vi "FestoCPX.Station.Prod.TakeAB.vi"(7 "SuckerID":i32, 8 "error in":errorcluster) -> (0 "error out":errorcluster, 1 "Slot":cluster{"A":bool, "B":bool}, 2 "Error reason B":T2, 3 "Error reason A":T2, 4 "Prod Present":T1)   [LabVIEW 2016]
uses:
  Sequence/Sequence.Test.BreakReason.ctl
  FestoCPX.Station.ProdPresent.ctl
  Station/Station.ValvePosition.ctl
  Station/Station.ProductSlot.ctl
  FestoCPX.Station.ProdArmPosition.ctl
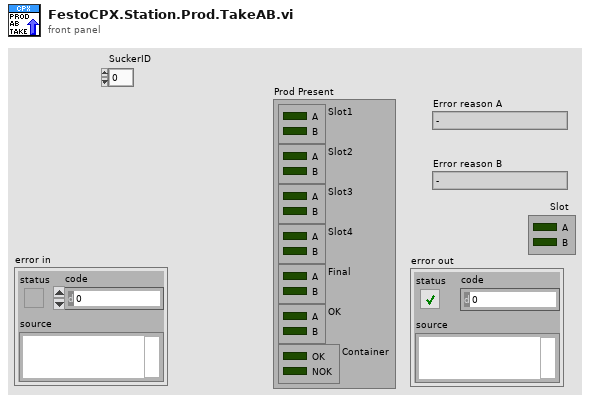
[diagram p1: front panel]
types:
  T1 = typedef "FestoCPX.Station.ProdPresent.ctl" = cluster{"Slot1":cluster{"A":bool, "B":bool}, "Slot2":cluster{"A":bool, "B":bool}, "Slot3":cluster{"A":bool, "B":bool}, "Slot4":cluster{"A":bool, "B":bool}, "Final":cluster{"A":bool, "B":bool}, "OK":cluster{"A":bool, "B":bool}, "Container":cluster{"OK":bool, "NOK":bool}}
  T2 = typedef "Sequence.Test.BreakReason.ctl" = enum16{"-", "NOK container", "OK container", "Rev empty", "Rev missing", "Rev wrong", "Fork missing", "Fork wrong", "NOK limit", "Unload failure", "Single slot", "Part done", "Err: Prod move work", "Err: Prod move home", "Err: Prod lift work", "Err: Prod lift home", "Err: Prod Arm Work", "Err: Prod Arm NOK", "Err: Prod Arm OK", "Err: Prod NOK suck", "Err: Prod NOK drop", "Err: Prod OK missing", "Err: Prod OK suck", "Err: Prod OK drop"}
  T3 = typedef "Station.ProductSlot.ctl" = enum8{"A", "B"}
  T4 = typedef "Station.ValvePosition.ctl" = enum16{"Home", "Work"}
  T5 = typedef "FestoCPX.Station.ProdArmPosition.ctl" = enum16{"Work", "OK", "NOK"}
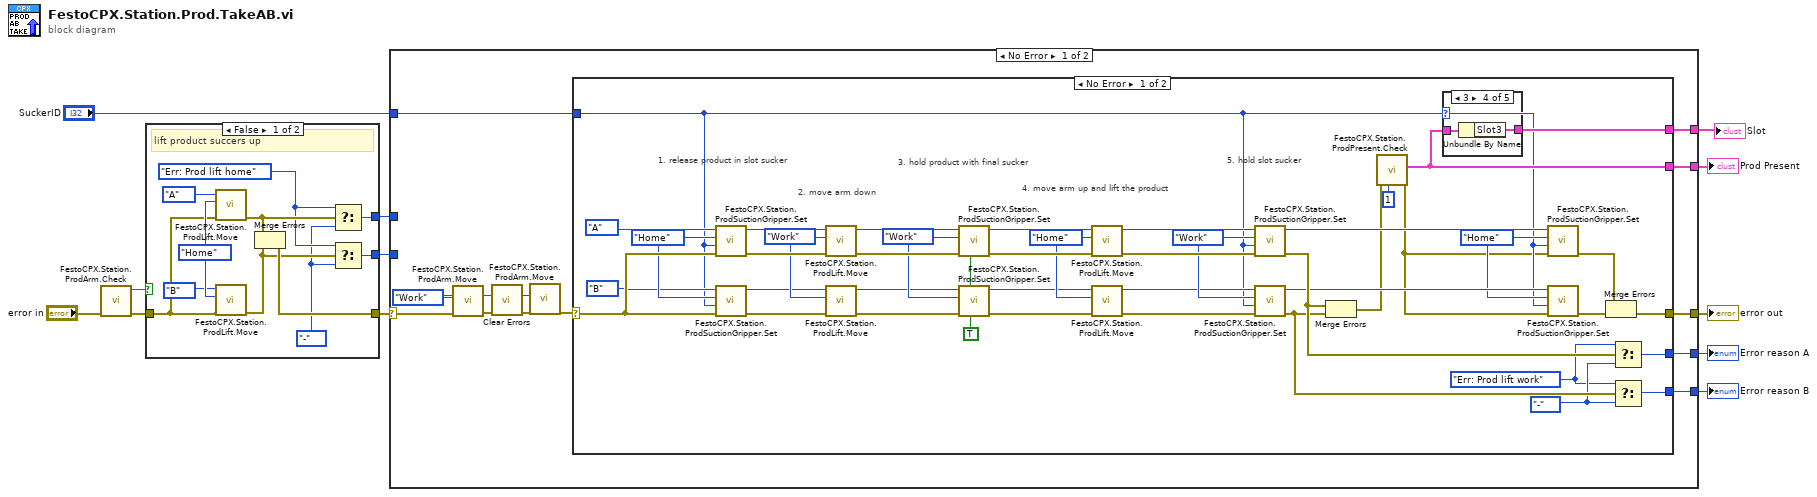
[diagram p0: block diagram]
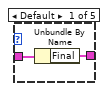
[diagram p2: hidden frame]
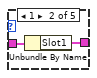
[diagram p3: hidden frame]
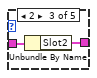
[diagram p4: hidden frame]
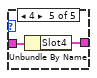
[diagram p5: hidden frame]
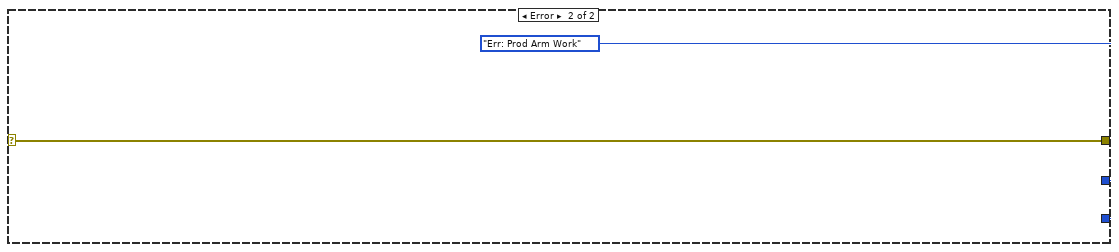
[diagram p6: hidden frame]
diagram:
  n1 = call "FestoCPX.Station.ProdArm.Check.vi"("error in"="error in") -> ("error out"=w12:errorcluster, "Work"=w11:bool)  [unwired: 6 in, 3 out]
  n2 = case shown="False" w11 {
    tunnel: w12 -> [w20 w24]
    tunnel: [w19 w24] -> w6
    tunnel: [w14 _] -> w10
    tunnel: [w13 _] -> w9
    frame False {
      w15 = Sequence.Test.BreakReason."-" ("Pause status")
      w16 = Sequence.Test.BreakReason."Err: Prod lift home" ("Pause status")
      w22 = Station.ValvePosition."Home" ("Position")
      # "lift product succers up"
      n3 = call "FestoCPX.Station.ProdLift.Move.vi"("error in"=w20, "Position"=w22, "Slot"=Station.ProductSlot."A") -> ("error out"=w18:errorcluster)  [unwired: 8 in]
      n4 = call "FestoCPX.Station.ProdLift.Move.vi"("error in"=w20, "Position"=w22, "Slot"=Station.ProductSlot."B") -> ("error out"=w17:errorcluster)  [unwired: 8 in]
      n5 = Merge Errors(w18, w17) -> (w19:errorcluster)
      n6 = Select(t=w16, s=w18, f=w15) -> (s? t:f=w14:T2)
      n7 = Select(t=w16, s=w17, f=w15) -> (s? t:f=w13:T2)
    }
    frame True {
      # "Arm already in work position"
    }
  }
  n8 = case shown="No Error" w6 {
    selector: w6 -> [w34 w81]
    tunnel: w10 -> [_ w83]
    tunnel: w9 -> [_ w82]
    tunnel: [w35 w83] -> w8
    tunnel: [w33 w82] -> w5
    tunnel: [w32 w81] -> w4
    tunnel: "SuckerID" -> [w31 _]
    tunnel: [w30 _] -> w2
    tunnel: [w29 _] -> w1
    frame No Error {
      w25 = FestoCPX.Station.ProdArmPosition."Work" ("Product Status")
      n9 = call "FestoCPX.Station.ProdArm.Move.vi"("error in"=w34, "Product Status"=w25) -> ("error out"=w28:errorcluster)  [unwired: 9 in]
      n10 = call <vilib>:"Clear Errors.vi"("error in (no error)"=w28) -> ("error out"=w27:errorcluster)  [unwired: 5 in, 1 out]
      n11 = call "FestoCPX.Station.ProdArm.Move.vi"("error in"=w27, "Product Status"=w25) -> ("error out"=w26:errorcluster)  [unwired: 9 in]
      n12 = case shown="No Error" w26 {
        selector: w26 -> [w62 w80]
        tunnel: [w51 w79] -> w35
        tunnel: [w52 w79] -> w33
        tunnel: [w40 w80] -> w32
        tunnel: w31 -> [w38 _]
        tunnel: [w48 _] -> w30
        tunnel: [w45 _] -> w29
        frame No Error {
          w39 = Station.ValvePosition."Home" ("Position")
          w46 = Sequence.Test.BreakReason."Err: Prod lift work" ("Pause status")
          w47 = Sequence.Test.BreakReason."-" ("Pause status")
          w54 = Station.ValvePosition."Work" ("Position")
          w57 = TRUE ("wait for product (F)")
          w59 = Station.ValvePosition."Work" ("Position")
          w61 = Station.ValvePosition."Home" ("Position")
          w58 = Station.ValvePosition."Home" ("Position")
          w60 = Station.ValvePosition."Work" ("Position")
          w43 = Station.ProductSlot."B" ("Slot")
          w44 = Station.ProductSlot."A" ("Slot")
          # "5. hold slot sucker"
          # "2. move arm down"
          # "4. move arm up and lift the product"
          # "3. hold product with final sucker"
          # "1. release product in slot sucker"
          n13 = call "FestoCPX.Station.ProdSuctionGripper.Set.vi"("error in"=w62, "Sucker (0: Final)"=w38, "Position"=w61, "Slot"=w44) -> ("error out"=w66:errorcluster)  [unwired: 6 in, 1 out]
          n14 = call "FestoCPX.Station.ProdSuctionGripper.Set.vi"("error in"=w62, "Sucker (0: Final)"=w38, "Position"=w61, "Slot"=w43) -> ("error out"=w65:errorcluster)  [unwired: 6 in, 1 out]
          n15 = call "FestoCPX.Station.ProdLift.Move.vi"("error in"=w66, "Position"=w60, "Slot"=w44) -> ("error out"=w67:errorcluster)  [unwired: 8 in]
          n16 = call "FestoCPX.Station.ProdLift.Move.vi"("error in"=w65, "Position"=w60, "Slot"=w43) -> ("error out"=w64:errorcluster)  [unwired: 8 in]
          n17 = call "FestoCPX.Station.ProdSuctionGripper.Set.vi"("wait for product (F)"=w57, "error in"=w67, "Position"=w59, "Slot"=w44) -> ("error out"=w68:errorcluster)  [unwired: 6 in, 1 out]
          n18 = call "FestoCPX.Station.ProdSuctionGripper.Set.vi"("wait for product (F)"=w57, "error in"=w64, "Position"=w59, "Slot"=w43) -> ("error out"=w63:errorcluster)  [unwired: 6 in, 1 out]
          n19 = call "FestoCPX.Station.ProdLift.Move.vi"("error in"=w68, "Position"=w58, "Slot"=w44) -> ("error out"=w56:errorcluster)  [unwired: 8 in]
          n20 = call "FestoCPX.Station.ProdLift.Move.vi"("error in"=w63, "Position"=w58, "Slot"=w43) -> ("error out"=w55:errorcluster)  [unwired: 8 in]
          n21 = call "FestoCPX.Station.ProdSuctionGripper.Set.vi"("error in"=w56, "Sucker (0: Final)"=w38, "Position"=w54, "Slot"=w44) -> ("error out"=w50:errorcluster)  [unwired: 6 in, 1 out]
          n22 = call "FestoCPX.Station.ProdSuctionGripper.Set.vi"("error in"=w55, "Sucker (0: Final)"=w38, "Position"=w54, "Slot"=w43) -> ("error out"=w49:errorcluster)  [unwired: 6 in, 1 out]
          n23 = Merge Errors(w50, w49) -> (w36:errorcluster)
          n24 = call "FestoCPX.Station.ProdPresent.Check.vi"("Stab Counter (0)"=1 ("Max Stab time [ms] (0)"), "error in"=w36) -> ("error out"=w37:errorcluster, "Prod Present"=w48:T1)  [unwired: 4 in, 4 out]
          n25 = case shown="3" w38 {
            tunnel: w48 -> [w70 w72 w74 w76 w78]
            tunnel: [w69 w71 w73 w75 w77] -> w45
            frame Default {
              n26 = Unbundle By Name(w70) -> ("Final"=w69:cluster{"A":bool, "B":bool})
            }
            frame 1 {
              n27 = Unbundle By Name(w72) -> ("Slot1"=w71:cluster{"A":bool, "B":bool})
            }
            frame 2 {
              n28 = Unbundle By Name(w74) -> ("Slot2"=w73:cluster{"A":bool, "B":bool})
            }
            frame 3 {
              n29 = Unbundle By Name(w76) -> ("Slot3"=w75:cluster{"A":bool, "B":bool})
            }
            frame 4 {
              n30 = Unbundle By Name(w78) -> ("Slot4"=w77:cluster{"A":bool, "B":bool})
            }
          }
          n31 = call "FestoCPX.Station.ProdSuctionGripper.Set.vi"("error in"=w37, "Sucker (0: Final)"=w38, "Position"=w39, "Slot"=w44) -> ("error out"=w42:errorcluster)  [unwired: 6 in, 1 out]
          n32 = call "FestoCPX.Station.ProdSuctionGripper.Set.vi"("error in"=w37, "Sucker (0: Final)"=w38, "Position"=w39, "Slot"=w43) -> ("error out"=w41:errorcluster)  [unwired: 6 in, 1 out]
          n33 = Merge Errors(w42, w41) -> (w40:errorcluster)
          n34 = Select(t=w46, s=w50, f=w47) -> (s? t:f=w51:T2)
          n35 = Select(t=w46, s=w49, f=w47) -> (s? t:f=w52:T2)
        }
        frame Error {
          w79 = Sequence.Test.BreakReason."Err: Prod Arm Work" ("Pause status")
        }
      }
    }
    frame Error {
    }
  }
  "Error reason A" <- w8
  "Error reason B" <- w5
  "error out" <- w4
  "Prod Present" <- w2
  "Slot" <- w1
